vi "FL_Segment_map_by_color.vi"(2 "Array of presence count in":u32[][](array[numeric]), 3 "Array of the segment to color correspondences":u32[][](array[numeric]), 4 "Array of the pixel to color correspondences":u32[][](array[numeric]), 5 "Mouse abs. coordinates, pix":T1) -> (0 "Array of presence count out":u32[][](array[numeric]), 1 "Current segment' number":u32)   [LabVIEW 2016]
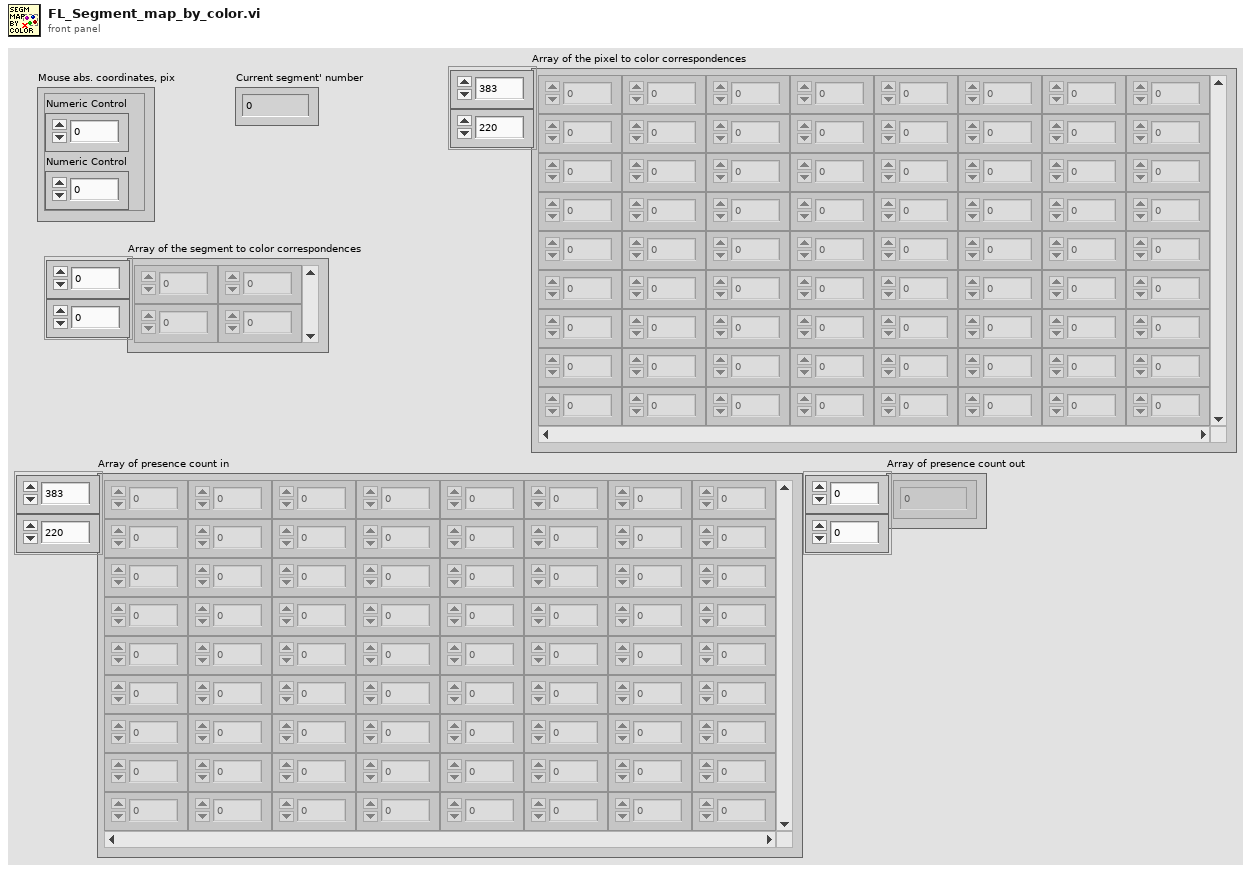
[diagram p1: front panel]
types:
  T1 = cluster{"Numeric Control":dbl, "Numeric Control":dbl}
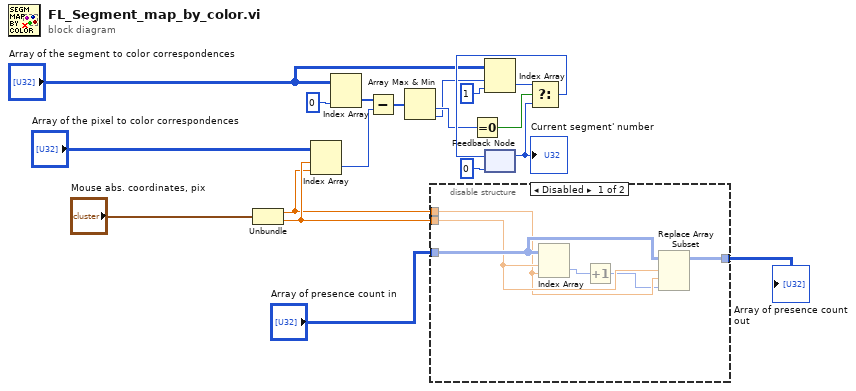
[diagram p0: block diagram]
diagram:
  n1 = Unbundle("Mouse abs. coordinates, pix") -> ("Numeric Control"=w2:dbl, "Numeric Control"=w3:dbl)
  n2 = Index Array(array="Array of the pixel to color correspondences", index (row)=w3, index (col)=w2) -> (element=w9:u32)
  n3 = Index Array(array="Array of the segment to color correspondences", index (col)=0 ("disabled index (col)")) -> (element=w8:u32[])  [unwired: 1 in]
  n4 = Subtract(x=w8, y=w9) -> (x-y=w10:u32[])
  n5 = Array Max & Min(array=w10) -> (min value=w14:u32, min index (indices)=w12:i32)  [unwired: 2 out]
  n6 = disable-structure shown="Disabled" {
    disable-tunnel: "Array of presence count in" -> [w24 _]
    disable-tunnel: w3 -> [w23 _]
    disable-tunnel: w2 -> [w22 _]
    disable-tunnel: [w20 _] -> w1
    frame Disabled {
      n7 = Index Array(array=w24, index (row)=w23, index (col)=w22) -> (element=w25:u32)
      n8 = Increment(x=w25) -> (x+1=w21:u32)
      n9 = Replace Array Subset(array=w24, new element=w21, index (row)=w23, index (col)=w22) -> (w20:u32[][])
    }
    frame Enabled {
    }
  }
  "Array of presence count out" <- w1
  n10 = Equal To 0?(x=w14) -> (x = 0?=w16:bool)
  n11 = Index Array(array="Array of the segment to color correspondences", index (row)=w12, index (col)=1 ("disabled index (col)")) -> (element=w15:u32)
  n12 = feedback #1(u32 0 ("Color for central segment")) -> (w18:u32)
  "Current segment' number" <- w18
  n13 = Select(t=w15, s=w16, f=w18) -> (s? t:f=w17:u32)
  n14 = feedback-in #1(w17) -> ()
